vi "ForLoop_Basic.vi"() -> ()   [LabVIEW 2018]
panel:
  out "x+1 2":i32
  out "x+1":i32
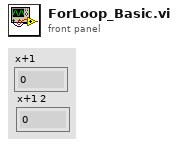
[diagram p1: front panel]
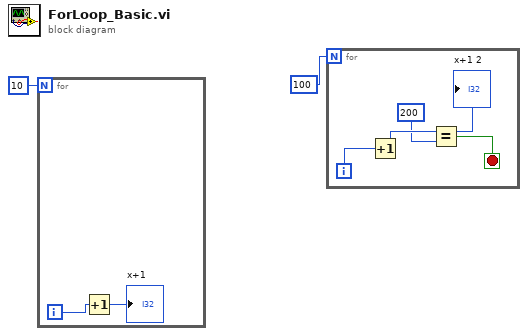
[diagram p0: block diagram]
diagram:
  n1 = for {
    N: 10 -> [_]
    i -> [w4]
    n2 = Increment(x=w4) -> (x+1=→"x+1":i32)
  }
  n3 = for {
    N: 100 -> [_]
    i -> [w7]
    stop <- w5 stop-if-true
    n4 = Increment(x=w7) -> (x+1=w8:i32)
    "x+1 2" <- w8
    n5 = Equal?(x=w8, y=200) -> (x = y?=w5:bool)
  }
